vi "CRYGet Category Name with MultiLang.vi"(11 "Category":string) -> (3 "Name":string)   [LabVIEW 2013]
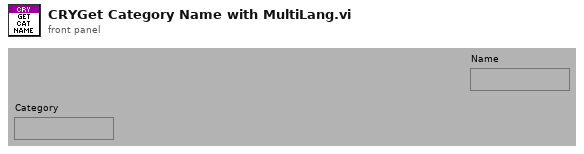
[diagram p1: front panel]
types:
  T1 = enum32{"English", "Chinese", "Korean", "Japanese", "Russian", "Chinese traditional"}
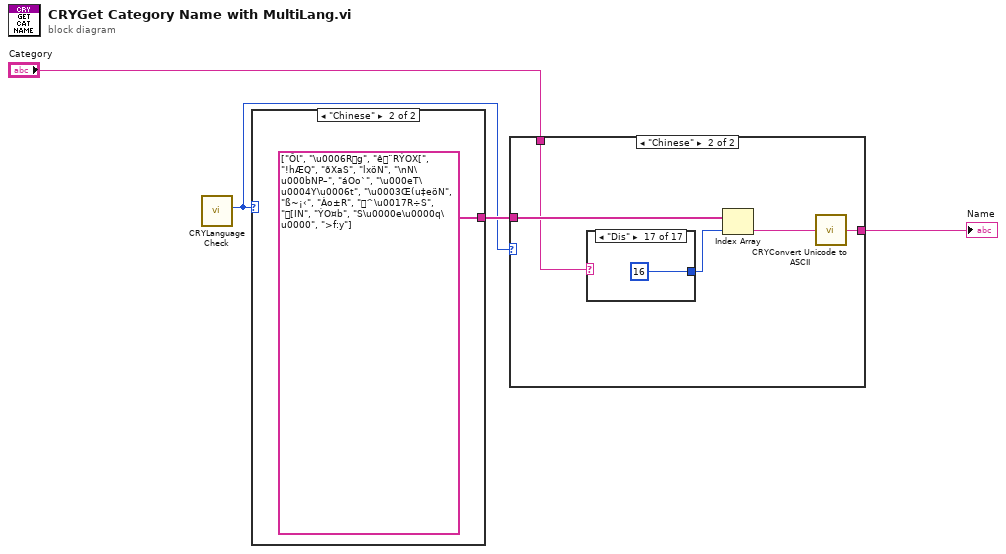
[diagram p0: block diagram]
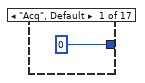
[diagram p3: hidden frame]
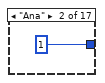
[diagram p4: hidden frame]
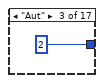
[diagram p5: hidden frame]
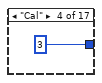
[diagram p6: hidden frame]
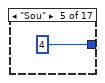
[diagram p7: hidden frame]
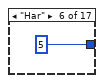
[diagram p8: hidden frame]
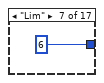
[diagram p9: hidden frame]
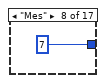
[diagram p10: hidden frame]
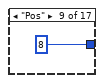
[diagram p11: hidden frame]
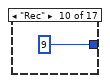
[diagram p12: hidden frame]
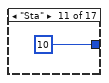
[diagram p13: hidden frame]
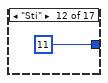
[diagram p14: hidden frame]
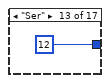
[diagram p15: hidden frame]
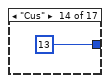
[diagram p16: hidden frame]
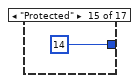
[diagram p17: hidden frame]
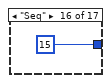
[diagram p18: hidden frame]
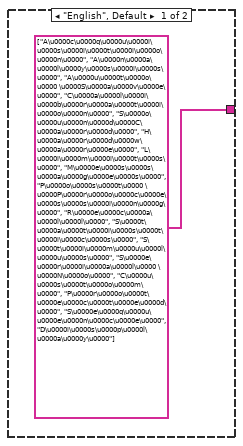
[diagram p19: hidden frame]
diagram:
  n1 = call "CRYLanguage Check.vi"() -> ("Language"=w1:T1)  [unwired: 10 in, 1 out]
  n2 = case shown="\"Chinese\"" w1 {
    tunnel: [string[] ["A\u0000c\u0000q\u0000u\u0000i\u0000s\u0000i\u0000t\u0000i\u0000o\u0000n\u0000", "A\u0000n\u0000a\u0000l\u0000y\u0000s\u0000i\u0000s\u0000", "A\u0000u\u0000t\u0000o\u0000 \u0000S\u0000a\u0000v\u0000e\u0000", "C\u0000a\u0000l\u0000i\u0000b\u0000r\u0000a\u0000t\u0000i\u0000o\u0000n\u0000", "S\u0000o\u0000u\u0000n\u0000d\u0000C\u0000a\u0000r\u0000d\u0000", "H\u0000a\u0000r\u0000d\u0000w\u0000a\u0000r\u0000e\u0000", "L\u0000i\u0000m\u0000i\u0000t\u0000s\u0000", "M\u0000e\u0000s\u0000s\u0000a\u0000g\u0000e\u0000s\u0000", "P\u0000o\u0000s\u0000t\u0000 \u0000P\u0000r\u0000o\u0000c\u0000e\u0000s\u0000s\u0000i\u0000n\u0000g\u0000", "R\u0000e\u0000c\u0000a\u0000l\u0000l\u0000", "S\u0000t\u0000a\u0000t\u0000i\u0000s\u0000t\u0000i\u0000c\u0000s\u0000", "S\u0000t\u0000i\u0000m\u0000u\u0000l\u0000u\u0000s\u0000", "S\u0000e\u0000r\u0000i\u0000a\u0000l\u0000 \u0000N\u0000o\u0000", "C\u0000u\u0000s\u0000t\u0000o\u0000m\u0000", "P\u0000r\u0000o\u0000t\u0000e\u0000c\u0000t\u0000e\u0000d\u0000", "S\u0000e\u0000q\u0000u\u0000e\u0000n\u0000c\u0000e\u0000", "D\u0000i\u0000s\u0000p\u0000l\u0000a\u0000y\u0000"] ("Array") string[] ["ǑƖ", "\u0006Rg", "ê¨RÝOX[", "!hÆQ", "ðXaS", "lxöN", "\nN\u000bNP–", "áOo`", "\u000eT\u0004Y\u0006t", "\u0003Œ(u‡eöN", "ß~¡‹", "Ào±R", "^\u0017R÷S", "ꁚ[IN", "ÝO¤b", "S\u0000e\u0000q\u0000", ">f:y"] ("Array")] -> w4
    frame "English", Default {
    }
    frame "Chinese" {
    }
  }
  n3 = case shown="\"Chinese\"" w1 {
    tunnel: w4 -> [_ w12]
    tunnel: "Category" -> [w7 w9]
    tunnel: [w7 w10] -> w2
    frame "English", Default {
    }
    frame "Chinese" {
      n4 = case shown="\"Dis\"" w9 {
        tunnel: [0 ("index") 1 ("index") 2 ("index") 3 ("index") 4 ("index") 5 ("index") 6 ("index") 7 ("index") 8 ("index") 9 ("index") 10 ("index") 11 ("index") 12 ("index") 13 ("index") 14 ("index") 15 ("index") 16 ("index")] -> w8
        frame "Acq", Default {
        }
        frame "Ana" {
        }
        frame "Aut" {
        }
        frame "Cal" {
        }
        frame "Sou" {
        }
        frame "Har" {
        }
        frame "Lim" {
        }
        frame "Mes" {
        }
        frame "Pos" {
        }
        frame "Rec" {
        }
        frame "Sta" {
        }
        frame "Sti" {
        }
        frame "Ser" {
        }
        frame "Cus" {
        }
        frame "Protected" {
        }
        frame "Seq" {
        }
        frame "Dis" {
        }
      }
      n5 = Index Array(array=w12, index=w8) -> (element=w11:string)
      n6 = call "CRYConvert Unicode to ASCII.vi"("Unicode"=w11) -> ("ASCII"=w10:string)  [unwired: 4 in]
    }
  }
  "Name" <- w2
